vi "PCP Last data GFV.vi"(1 "Action(GET)":enum16{"GET", "SET"}(ring), 7 "PCP Data in":T1, 11 "error in (no error)":errorcluster) -> (6 "ms since last data":u32, 8 "PCP Data out":T1, 15 "error out":errorcluster)   [LabVIEW 2011]
uses:
  PCP return data types/RDd return.ctl
  PCP return data types/RA return Analog I.ctl
  PCP return data types/RP return digital IO.ctl
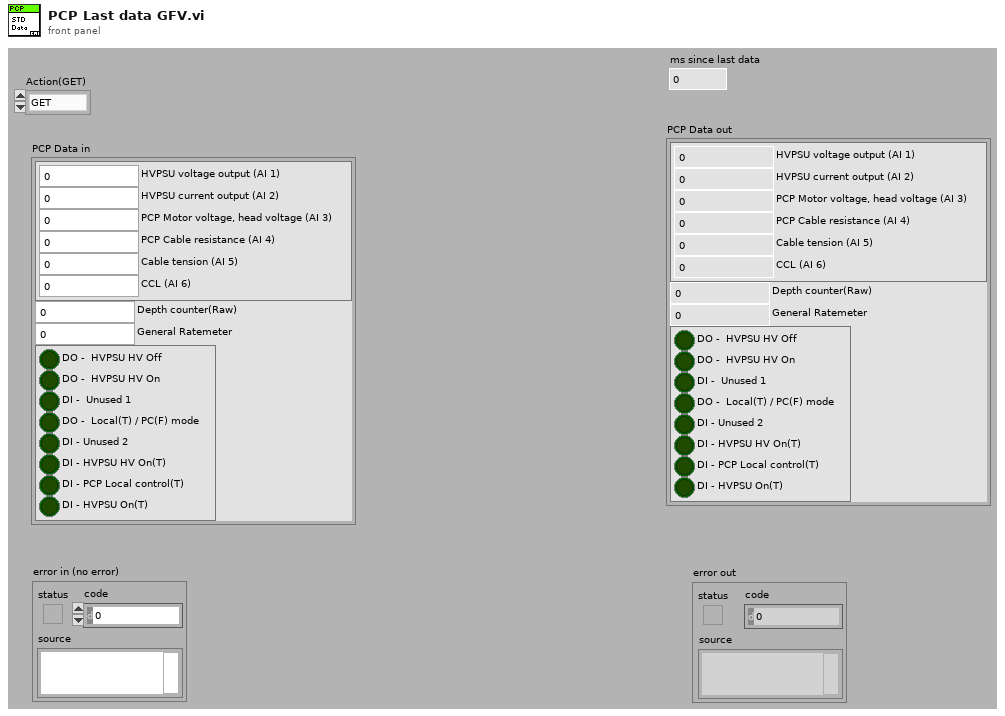
[diagram p1: front panel]
types:
  T1 = typedef "RDd return.ctl" = cluster{"AI":T2, "Depth counter(Raw)":i32, "General Ratemeter":dbl, "Digital ports":T3}
  T2 = typedef "RA return Analog I.ctl" = cluster{"HVPSU voltage output (AI 1)":dbl, "HVPSU current output (AI 2)":dbl, "PCP Motor voltage, head voltage (AI 3)":dbl, "PCP Cable resistance (AI 4)":dbl, "Cable tension (AI 5)":dbl, "CCL (AI 6)":dbl}
  T3 = typedef "RP return digital IO.ctl" = cluster{"DO -  HVPSU HV Off":bool, "DO -  HVPSU HV On":bool, "DI -  Unused 1":bool, "DO -  Local(T) / PC(F) mode":bool, "DI - Unused 2":bool, "DI - HVPSU HV On(T)":bool, "DI - PCP Local control(T)":bool, "DI - HVPSU On(T)":bool}
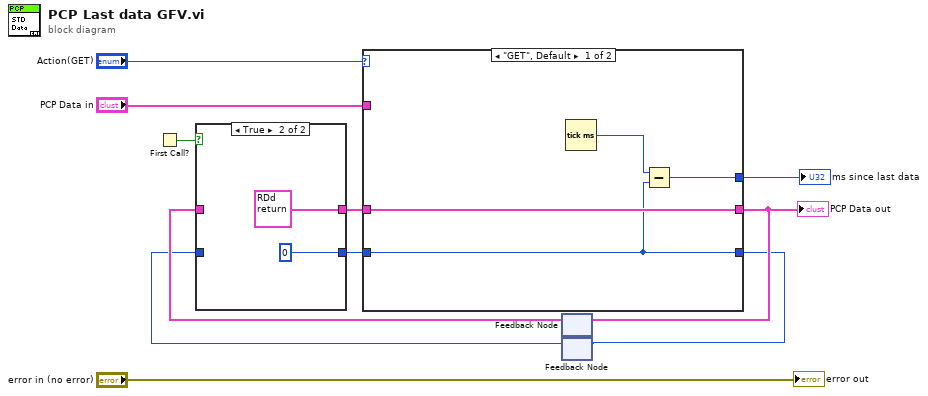
[diagram p0: block diagram]
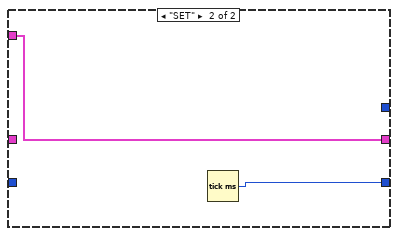
[diagram p3: hidden frame]
diagram:
  n1 = First Call?() -> (First Call?: T/F=w8:bool)
  n2 = feedback #1() -> (w9:T1)  [unwired: 1 in]
  n3 = feedback #2() -> (w2:u32)  [unwired: 1 in]
  n4 = case shown="True" w8 {
    tunnel: w9 -> [w13 _]
    tunnel: [w13 T1 {"AI"={"HVPSU voltage output (AI 1)"=nan, "HVPSU current output (AI 2)"=nan, "PCP Motor voltage, head voltage (AI 3)"=nan, "PCP Cable resistance (AI 4)"=nan, "Cable tension (AI 5)"=nan, "CCL (AI 6)"=nan}, "Depth counter(Raw)"=0, "General Ratemeter"=nan, "Digital ports"={"DO -  HVPSU HV Off"=FALSE, "DO -  HVPSU HV On"=FALSE, "DI -  Unused 1"=FALSE, "DO -  Local(T) / PC(F) mode"=FALSE, "DI - Unused 2"=FALSE, "DI - HVPSU HV On(T)"=FALSE, "DI - PCP Local control(T)"=FALSE, "DI - HVPSU On(T)"=FALSE}} ("PCP Data")] -> w6
    tunnel: [w12 u32 0 ("millisecond timer value")] -> w4
    tunnel: w2 -> [w12 _]
    frame False {
    }
    frame True {
    }
  }
  n5 = case shown="\"GET\", Default" "Action(GET)" {
    tunnel: [w19 w21] -> w7
    tunnel: w6 -> [w19 _]
    tunnel: "PCP Data in" -> [_ w21]
    tunnel: w4 -> [w17 _]
    tunnel: [w17 w20] -> w3
    tunnel: [w16 _] -> w1
    frame "GET", Default {
      n6 = Tick Count (ms)() -> (millisecond timer value=w18:u32)
      n7 = Subtract(x=w18, y=w17) -> (x-y=w16:u32)
    }
    frame "SET" {
      n8 = Tick Count (ms)() -> (millisecond timer value=w20:u32)
    }
  }
  "PCP Data out" <- w7
  "ms since last data" <- w1
  n9 = feedback-in #1(w7) -> ()
  n10 = feedback-in #2(w3) -> ()
  "error out" <- "error in (no error)"
